vi "SaveImage.vi"(8 "Error In":errorcluster, 10 "Image In":T1[](array[typedef]), 11 "Snapshot images folder path":path) -> (0 "Error Out":errorcluster)   [LabVIEW 2017]
uses:
  <vilib>/vision/Image Controls.llb/IMAQ Image.ctl
  <vilib>/vision/NI_Vision_Development_Module.lvlib
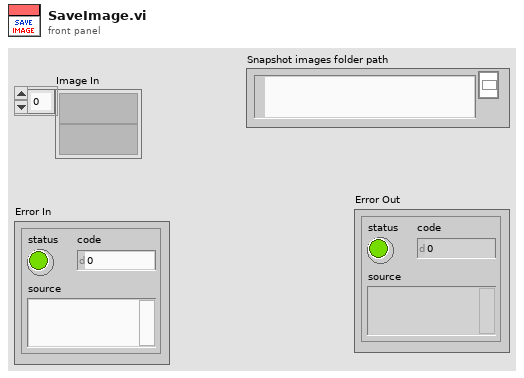
[diagram p1: front panel]
types:
  T1 = typedef "IMAQ Image.ctl" = refnum<image>
  T2 = typedef "Image Type" = u32
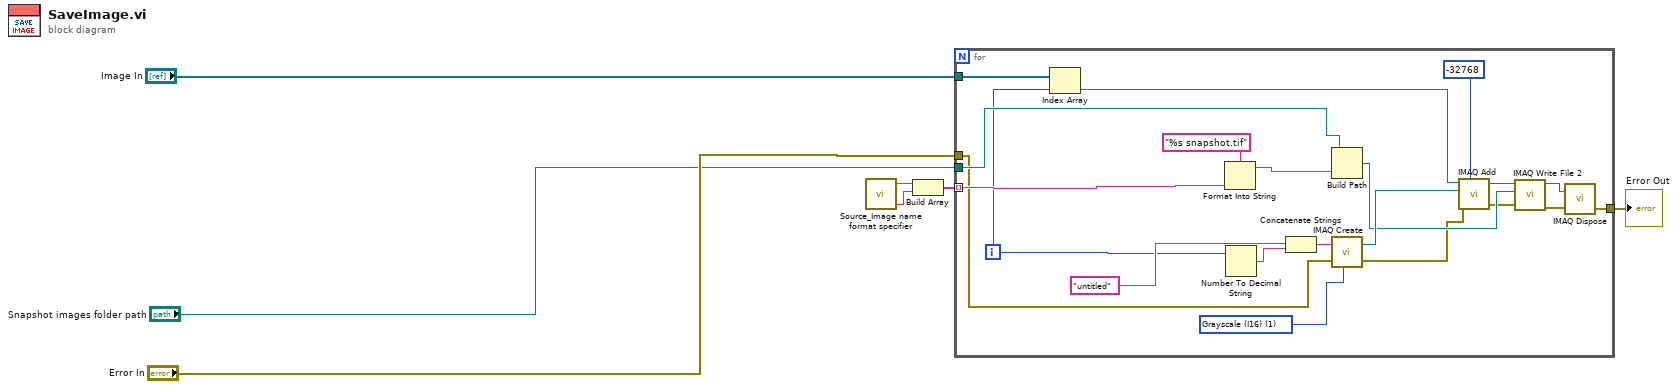
[diagram p0: block diagram]
diagram:
  n1 = call "Source_Image name format specifier.vi"() -> ("Red channel name"=w4:string, "Green channel name"=w3:string)  [unwired: 5 in, 1 out]
  n2 = Build Array(w4, w3) -> (w5:string[])
  n3 = for {
    tunnel: "Snapshot images folder path" -> [w16]
    tunnel: "Error In" -> [w15]
    tunnel: "Image In" -> [w12]
    tunnel: w5 -> [w26] mode=indexing
    tunnel: [w17] -> w6
    i -> [w9]
    w28 = T2 1 items=["Grayscale (U8)", "Grayscale (I16)", "Grayscale (SGL)", "Complex (CSG)", "RGB (U32)", "HSL (U32)", "RGB (U64)"] ("Image Type")
    n4 = Index Array(array=w12, index=w9) -> (element=w11:T1)
    n5 = Format Into String(format string="%s snapshot.tif", w26) -> (resulting string=w24:string)  [unwired: 2 in, 1 out]
    n6 = Number To Decimal String(number=w9) -> (decimal integer string=w21:string)  [unwired: 1 in]
    n7 = Concatenate Strings("untitled" ("Image Name"), w21) -> (w20:string)
    n8 = Build Path(base path=w16, name or relative path=w24) -> (appended path=w25:path)
    n9 = call "IMAQ Create"("Image Name"=w20, "Image Type"=w28, "error in (no error)"=w15) -> ("New Image"=w27:T1, "error out"=w14:errorcluster)  [unwired: 2 in]
    n10 = call "IMAQ Add"("Image Src A"=w11, "Constant"=i16 -32768, "Image Dst"=w27, "error in (no error)"=w14) -> ("Image Dst Out"=w23:T1, "error out"=w13:errorcluster)  [unwired: 3 in]
    n11 = call-poly "IMAQ Write File 2"("error in (no error)"=w13, "File Path"=w25, "Image"=w23) -> ("error out"=w18:errorcluster, "Image Out (duplicate)"=w19:T1)  [unwired: 7 in]
    n12 = call "IMAQ Dispose"("Image"=w19, "error in (no error)"=w18) -> ("error out"=w17:errorcluster)  [unwired: 4 in]
  }
  "Error Out" <- w6
